vi "Drive Handler.vi"(11 "JoystickDevRef":T1) -> ()   [LabVIEW 2019]
uses:
  <vilib>/Rock Robotics/WPI/Joystick/WPI_JoystickDevRef.ctl
  <vilib>/Rock Robotics/WPI/Joystick/WPI_JoystickDeviceEnum.ctl
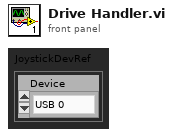
[diagram p1: front panel]
types:
  T1 = typedef "WPI_JoystickDevRef.ctl" = cluster{"Device":T2}
  T2 = typedef "WPI_JoystickDeviceEnum.ctl" = enum16{"USB 0", "USB 1", "USB 2", "USB 3", "USB 4", "USB 5"}
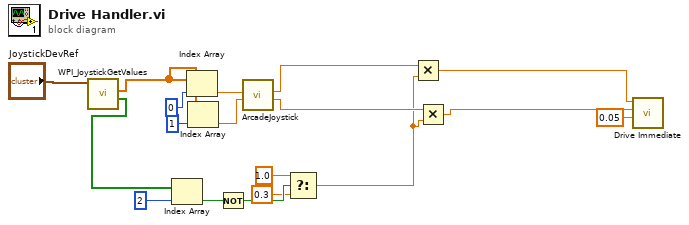
[diagram p0: block diagram]
diagram:
  n1 = call <vilib>:"WPI_JoystickGetValues.vi"("JoystickDevRef"="JoystickDevRef") -> ("Buttons"=w12:bool[], "Axes"=w15:dbl[])  [unwired: 6 in, 3 out]
  n2 = Index Array(array=w12, index=2) -> (element=w10:bool)
  n3 = Index Array(array=w15, index=0) -> (element=w14:dbl)
  n4 = Index Array(array=w15, index=1) -> (element=w13:dbl)
  n5 = Not(x=w10) -> (.not. x?=w7:bool)
  n6 = call "ArcadeJoystick.vi"("Y axis value"=w13, "X axis value"=w14) -> ("Right Motor Value"=w8:dbl, "Left Motor Value"=w9:dbl)  [unwired: 8 in]
  n7 = Select(t=1.0, s=w7, f=0.3) -> (s? t:f=w6:dbl)
  n8 = Multiply(x=w9, y=w6) -> (x*y=w4:dbl)
  n9 = Multiply(x=w8, y=w6) -> (x*y=w5:dbl)
  n10 = call "Drive Immediate.vi"("Deadband Value"=0.05, "Right Setpoint"=w5, "Left Setpoint"=w4) -> ()  [unwired: 8 in, 1 out]
